vi "Read Child Attributes Map.vi"(11 "TEMPLATE Actor in":refnum<class "TEMPLATE Actor.lvclass">) -> (2 "Child Attributes Map":T1)   [LabVIEW 2020, in "_Template.lvlib" / "Templates.lvlib" / "TEMPLATE jettl Actor.lvlib" / "TEMPLATE Actor.lvlib" / "TEMPLATE Actor.lvclass"]
uses:
  TEMPLATE Actor.lvclass
  TEMPLATE Actor.lvclass/TEMPLATE Actor.ctl
  jettl/jettl/Msg/Msg.lvclass
  jettl/jettl/Actor/Actor.lvclass
  jettl/jettl/Refs/Refs.lvclass
  jettl/jettl/Child Actor Attributes Map.ctl
  jettl/jettl/jettl.lvlib
  jettl/jettl/Transport/Transport.lvclass
  jettl/jettl/Actor Attributes.ctl
  jettl/jettl/Msgs.ctl
  jettl/jettl/Msg Names.ctl
  jettl/jettl/Unified Layer.ctl
panel:
  # "This front panel should not be manipulated."
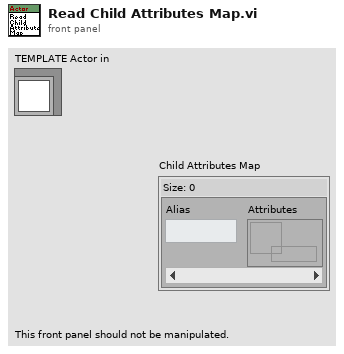
[diagram p1: front panel]
types:
  T1 = typedef "jettl.lvlib/Child Actor Attributes Map.ctl" = map{string, refnum<data-value>}
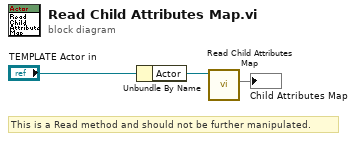
[diagram p0: block diagram]
diagram:
  # "This is a Read method and should not be further manipulated."
  n1 = Unbundle By Name("TEMPLATE Actor in") -> ("Actor"=w2:refnum<data-value>)
  n2 = call-dynamic "Read Child Attributes Map.vi"("Actor in"=w2) -> ("Child Attributes Map"=→"Child Attributes Map":T1)  [unwired: 10 in]
